vi "Begin.vi"(8 "error in":errorcluster) -> (0 "error out":errorcluster)   [LabVIEW 2016]
doc: "Called before other user functions, this VI is expected to open initial I/O refnums, load in file data, and do all program initialization. Notice that the <B>error out</B> terminal is simply used for data flow. Wiring it to other structures or subVIs ensures that this VI runs first."
uses:
  <vilib>/Rock Robotics/WPI/DriverStation/WPI_DriverStationRobotMode2.ctl
  <vilib>/Rock Robotics/WPI/Joystick/WPI_JoystickDeviceEnum.ctl
  <vilib>/Rock Robotics/WPI/ThirdParty/CanMotor/TalonSRX/WPI_CANTalonSRX_APIControlMode.ctl
  <vilib>/Rock Robotics/WPI/SafetyOutput/WPI_SafetyOutputConfigMenu.ctl
  <vilib>/Rock Robotics/SystemInterfaces/DIO/FPGA_DIOPWMChannel.ctl
  <vilib>/Rock Robotics/SystemInterfaces/DIO/FPGA_DIOChannel.ctl
  <vilib>/Rock Robotics/WPI/ThirdParty/CanMotor/TalonSRX/WPI_CANTalonSRX_Params.ctl
  Robot Global Data.vi
  <vilib>/Rock Robotics/Network Tables/NT Write String Array.vi
  <vilib>/Rock Robotics/WPI/MotorControl/WPI_MotorControlOpen TalonSRX.vi
  <vilib>/Rock Robotics/WPI/MotorControl/WPI_MotorControlOpen Talon.vi
  <vilib>/Rock Robotics/WPI/RobotDrive/WPI_RobotDriveOpen4MotorWithExistingMotors.vi
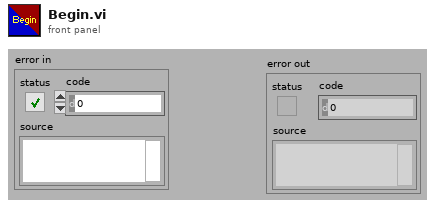
[diagram p1: front panel]
types:
  T1 = typedef "WPI_CANTalonSRX_Params.ctl" = u8
  T2 = typedef "WPI_CANTalonSRX_APIControlMode.ctl" = enum8{"Percent VBus", "Speed", "Position", "Slave", "Unchanged / Invalid", "Voltage Compensation", "Current", "Motion Profile", "Motion Magic"}
  T3 = typedef "FPGA_DIOPWMChannel.ctl" = enum8{"PWM 0", "PWM 1", "PWM 2", "PWM 3", "PWM 4", "PWM 5", "PWM 6", "PWM 7", "PWM 8", "PWM 9", "PWM MXP 0", "PWM MXP 1", "PWM MXP 2", "PWM MXP 3", "PWM MXP 4", "PWM MXP 5", "PWM MXP 6", "PWM MXP 7", "PWM MXP 8", "PWM MXP 9", "Invalid"}
  T4 = typedef "FPGA_DIOChannel.ctl" = enum8{"DIO 0", "DIO 1", "DIO 2", "DIO 3", "DIO 4", "DIO 5", "DIO 6", "DIO 7", "DIO 8", "DIO 9", "DIO MXP 0", "DIO MXP 1", "DIO MXP 2", "DIO MXP 3", "DIO MXP 4", "DIO MXP 5", "DIO MXP 6", "DIO MXP 7", "DIO MXP 8", "DIO MXP 9", "DIO MXP 10", "DIO MXP 11", "DIO MXP 12", "DIO MXP 13", "DIO MXP 14", "DIO MXP 15", "SPI Port CS1", "SPI Port CS2", "SPI Port CS3", "SPI Port MISO", "SPI Port MOSI", "Invalid"}
  T5 = typedef "WPI_JoystickDeviceEnum.ctl" = enum16{"USB 0", "USB 1", "USB 2", "USB 3", "USB 4", "USB 5"}
  T6 = typedef "WPI_SafetyOutputConfigMenu.ctl" = enum16{"Enable", "Disable"}
  T7 = typedef "WPI_DriverStationRobotMode2.ctl" = enum16{"Autonomous Disabled", "Autonomous Enabled", "Teleop Disabled", "Teleop Enabled", "Disconnected", "Finish", "Test Disabled", "Test Enabled", "Emergency Stopped"}
  T8 = typedef "WPI_DigitalInputDevRef.ctl" = cluster{"DevStatus":errorcluster, "DIO Channel":T4}
  T9 = typedef "WPI_MotorControlDeviceRef.ctl" = cluster{"DeviceStatus":errorcluster, "Type":T10, "PWM":cluster{"PWM Channel":T3, "DeadBand":T11}, "CAN":cluster{"Device Number":u8, "SetOutput VI Ref":variant, "GetOutput VI Ref":variant, "Enable VI Ref":variant, "Disable VI Ref":variant, "Data":variant}, "Invert":bool}
  T10 = typedef "WPI_MotorControlType.ctl" = enum16{"PWM", "CAN"}
  T11 = typedef "WPI_PWMDeadband.ctl" = cluster{"Name":string, "maxPositivePwm":i32, "minPositivePwm":i32, "centerPwm":i32, "maxNegativePwm":i32, "minNegativePwm":i32, "angularRange":u16}
  T12 = typedef "WPI_JoystickDevRef.ctl" = cluster{"Device":T5}
  T13 = typedef "WPI_RobotDriveDevRef.ctl" = cluster{"DevStatus":errorcluster, "Motors[]":T9[], "Square Inputs":bool, "Max Output":dbl}
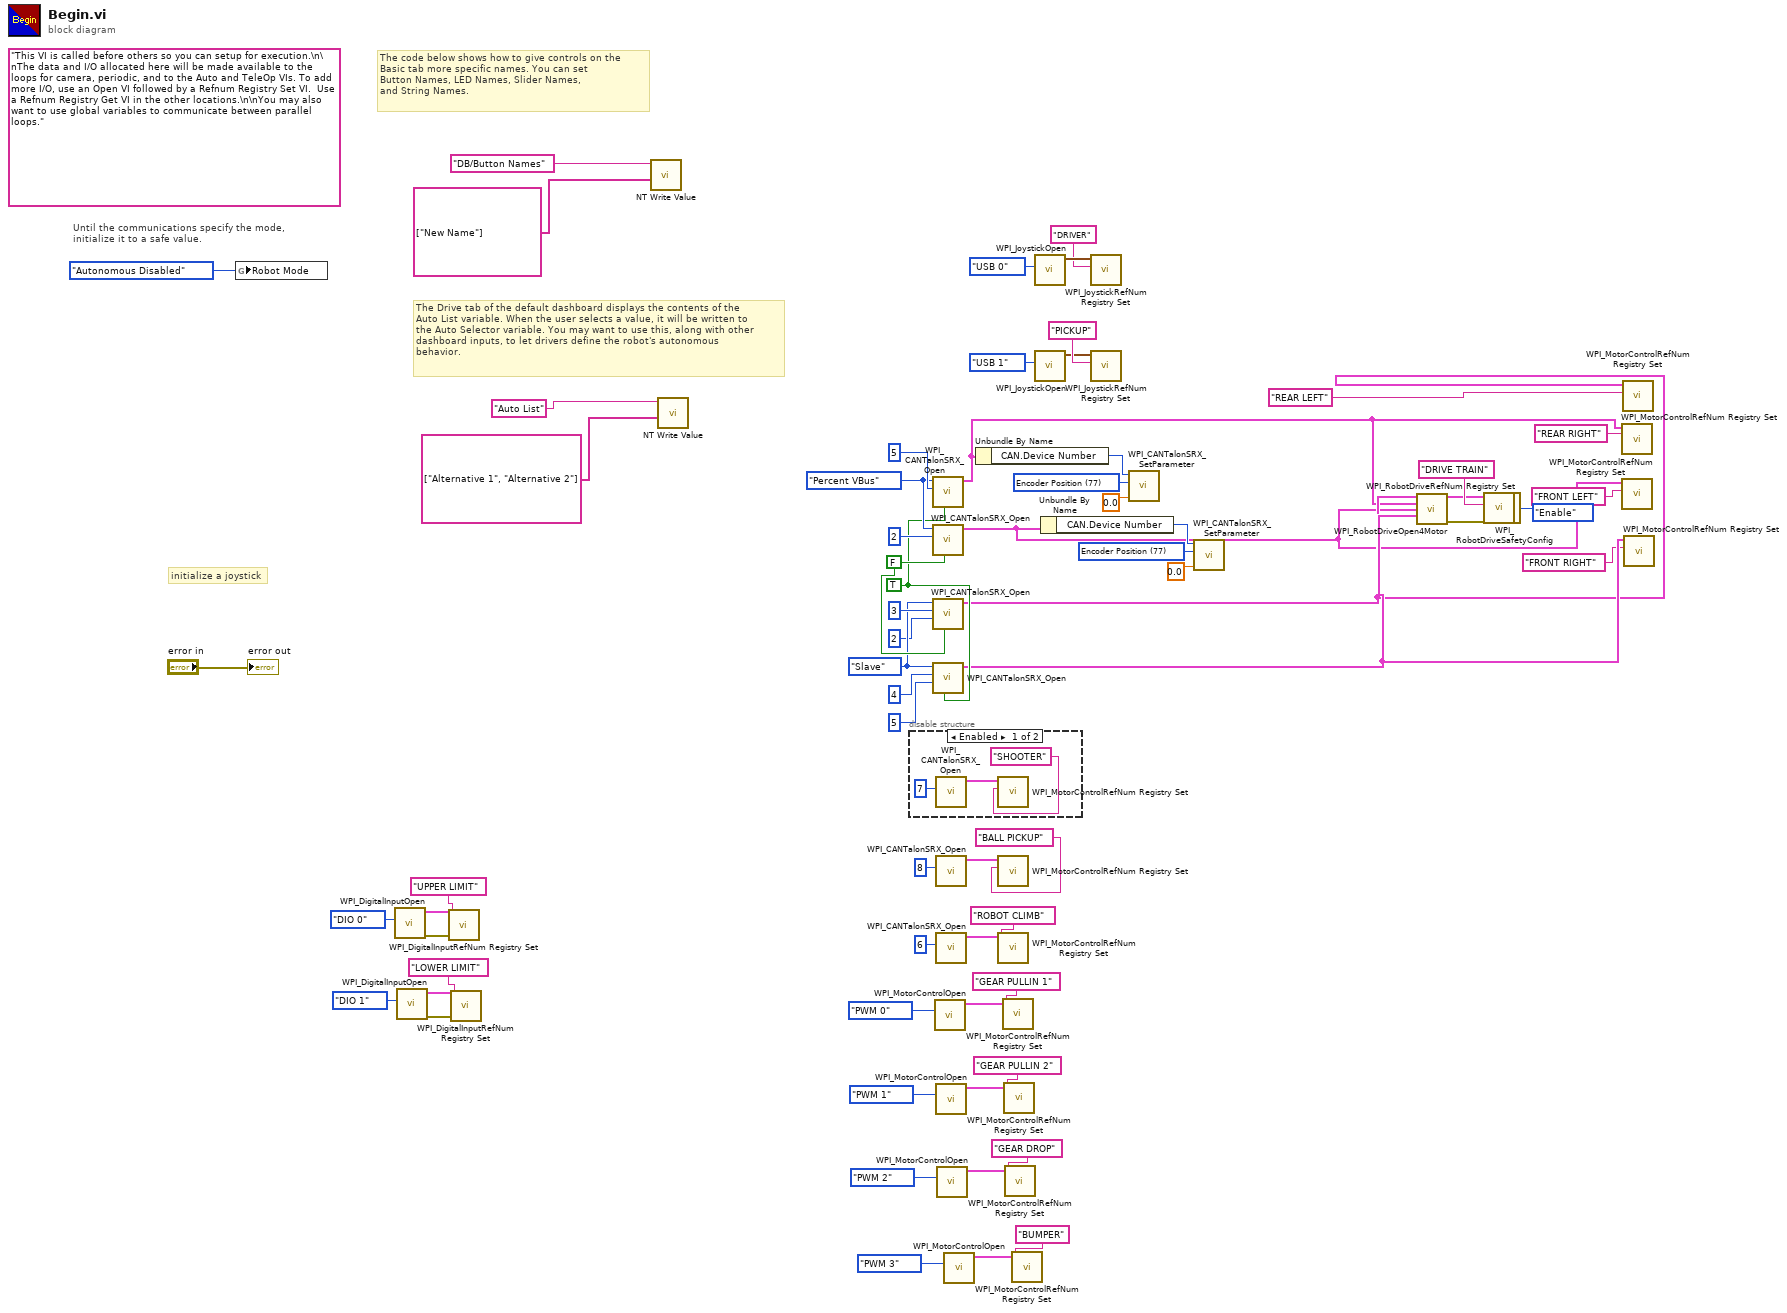
[diagram p0: block diagram]
diagram:
  w3 = T1 77 items=["Slot 0 - P"=1, "Slot 0 - I"=2, "Slot 0 - D"=3, "Slot 0 - F"=4, "Slot 0 - I Zone"=5, "Slot 0 - Ramp Rate"=6, "Slot 1 - P"=11, "Slot 1 - I"=12, "Slot 1 - D"=13, "Slot 1 - F"=14, "Slot 1 - I Zone"=15, "Slot 1 - Ramp Rate"=16, "Soft Limit - Forward"=21, "Soft Limit - Reverse"=22, "Soft Limit - Forward Enable"=23, "Soft Limit - Reverse Enable"=24, "On Boot - Brake Mode"=31, "On Boot - Limit Normally Closed - Forward"=32, "On Boot - Limit Normally Closed - Reverse"=33, "On Boot - Limit Disabled - Forward"=34, "On Boot - Limit Disabled - Reverse"=35, "Fault - Over Temp"=41, "Fault - Under Voltage"=42, "Fault - Forward Limit"=43, "Fault - Reverse Limit"=44, "Fault - Hardware Failure"=45, "Fault - Forward Soft Limit"=46, "Fault - Reverse Soft Limit"=47, "Sticky Fault - Over Temp"=48, "Sticky Fault - Under Voltage"=49, "Sticky Fault - Forward Limit"=50, "Sticky Fault - Reverse Limit"=51, "Sticky Fault - Forward Soft Limit"=52, "Sticky Fault - Reverse Soft Limit"=53, "Applied Throttle"=61, "Closed-Loop Error"=62, "Select Feedback Device"=63, "Reverse Closed-Loop Output"=64, "Mode Select"=65, "Profile Slot Select"=66, "Ramp Throttle"=67, "Reverse Feedback Sensor"=68, "Limit Switch Enabled"=69, "Limit Switch Closed - Forward"=70, "Limit Switch Closed - Reverse"=71, "Sensor Position"=73, "Sensor Velocity"=74, "Current"=75, "Brake is Enabled"=76, "Encoder Position"=77, "Encoder Velocity"=78, "Encoder Index Rise Events"=79, "Encoder A Pin State"=80, "Encoder B Pin State"=81, "Encoder Index Pin State"=82, "Analog In with Overflow"=83, "Analog In Velocity"=84, "Temperature"=85, "Battery Voltage"=86, "Reset Count"=87, "Reset Flags"=88, "Firmware Version"=89, "Settings Changed"=90, "Quad Filter Enable"=91, "Ignore Disable Broadcast"=92, "I Accumulator"=93, "Status 1 Frame Rate Ms"=94, "Status 2 Frame Rate Ms"=95, "Status 3 Frame Rate Ms"=96, "Status 4 Frame Rate Ms"=97, "Status 6 Frame Rate Ms"=98, "Status 7 Frame Rate Ms"=99, "Enable Index Pin Clear Position"=100, "Peak Positive Output"=104, "Nominal Positive Output"=105, "Peak Negative Output"=106, "Nominal Negative Output"=107, "Quad Index Pin Polarity"=108, "Status 8 Frame Rate Ms"=109, "Allow Position Overflow"=110, "Slot 0 - Allowable Closed-Loop Error"=111, "Number Potentiometer Turns"=112, "Encoder Codes Per Rev"=113, "Pulse Width Decoded Position"=114, "Analog Position"=115, "Voltage Compensation Rate (V/s)"=116, "Slot 1 - Allowable Closed-Loop Error"=117, "Motion Profile Has Underrun Err"=119, "Reserved 120"=120, "Legacy Control Mode"=121, "Motion Magic Acceleration"=122, "Motion Magic Cruise Velocity"=123, "Status 10 Frame Rate"=124, "Current Limit Threshold"=125, "CustomParam0"=137, "CustomParam1"=138, "PersStorageSaving"=139, "ClearPositionOnLimitF"=144, "ClearPositionOnLimitR"=145, "NominalBatteryVoltage"=146, "SampleVelocityPeriod"=147, "SampleVelocityWindow"=148] ("Parameter")
  w7 = T1 77 items=["Slot 0 - P"=1, "Slot 0 - I"=2, "Slot 0 - D"=3, "Slot 0 - F"=4, "Slot 0 - I Zone"=5, "Slot 0 - Ramp Rate"=6, "Slot 1 - P"=11, "Slot 1 - I"=12, "Slot 1 - D"=13, "Slot 1 - F"=14, "Slot 1 - I Zone"=15, "Slot 1 - Ramp Rate"=16, "Soft Limit - Forward"=21, "Soft Limit - Reverse"=22, "Soft Limit - Forward Enable"=23, "Soft Limit - Reverse Enable"=24, "On Boot - Brake Mode"=31, "On Boot - Limit Normally Closed - Forward"=32, "On Boot - Limit Normally Closed - Reverse"=33, "On Boot - Limit Disabled - Forward"=34, "On Boot - Limit Disabled - Reverse"=35, "Fault - Over Temp"=41, "Fault - Under Voltage"=42, "Fault - Forward Limit"=43, "Fault - Reverse Limit"=44, "Fault - Hardware Failure"=45, "Fault - Forward Soft Limit"=46, "Fault - Reverse Soft Limit"=47, "Sticky Fault - Over Temp"=48, "Sticky Fault - Under Voltage"=49, "Sticky Fault - Forward Limit"=50, "Sticky Fault - Reverse Limit"=51, "Sticky Fault - Forward Soft Limit"=52, "Sticky Fault - Reverse Soft Limit"=53, "Applied Throttle"=61, "Closed-Loop Error"=62, "Select Feedback Device"=63, "Reverse Closed-Loop Output"=64, "Mode Select"=65, "Profile Slot Select"=66, "Ramp Throttle"=67, "Reverse Feedback Sensor"=68, "Limit Switch Enabled"=69, "Limit Switch Closed - Forward"=70, "Limit Switch Closed - Reverse"=71, "Sensor Position"=73, "Sensor Velocity"=74, "Current"=75, "Brake is Enabled"=76, "Encoder Position"=77, "Encoder Velocity"=78, "Encoder Index Rise Events"=79, "Encoder A Pin State"=80, "Encoder B Pin State"=81, "Encoder Index Pin State"=82, "Analog In with Overflow"=83, "Analog In Velocity"=84, "Temperature"=85, "Battery Voltage"=86, "Reset Count"=87, "Reset Flags"=88, "Firmware Version"=89, "Settings Changed"=90, "Quad Filter Enable"=91, "Ignore Disable Broadcast"=92, "I Accumulator"=93, "Status 1 Frame Rate Ms"=94, "Status 2 Frame Rate Ms"=95, "Status 3 Frame Rate Ms"=96, "Status 4 Frame Rate Ms"=97, "Status 6 Frame Rate Ms"=98, "Status 7 Frame Rate Ms"=99, "Enable Index Pin Clear Position"=100, "Peak Positive Output"=104, "Nominal Positive Output"=105, "Peak Negative Output"=106, "Nominal Negative Output"=107, "Quad Index Pin Polarity"=108, "Status 8 Frame Rate Ms"=109, "Allow Position Overflow"=110, "Slot 0 - Allowable Closed-Loop Error"=111, "Number Potentiometer Turns"=112, "Encoder Codes Per Rev"=113, "Pulse Width Decoded Position"=114, "Analog Position"=115, "Voltage Compensation Rate (V/s)"=116, "Slot 1 - Allowable Closed-Loop Error"=117, "Motion Profile Has Underrun Err"=119, "Reserved 120"=120, "Legacy Control Mode"=121, "Motion Magic Acceleration"=122, "Motion Magic Cruise Velocity"=123, "Status 10 Frame Rate"=124, "Current Limit Threshold"=125, "CustomParam0"=137, "CustomParam1"=138, "PersStorageSaving"=139, "ClearPositionOnLimitF"=144, "ClearPositionOnLimitR"=145, "NominalBatteryVoltage"=146, "SampleVelocityPeriod"=147, "SampleVelocityWindow"=148] ("Parameter")
  w11 = WPI_CANTalonSRX_APIControlMode."Slave" ("Control Mode")
  w49 = TRUE ("Invert")
  w50 = FALSE ("Invert")
  w54 = WPI_CANTalonSRX_APIControlMode."Percent VBus" ("Control Mode")
  (unwired) "This VI is called before others so you can setup for execution.\n\nThe data and I/O allocated here will be made available to the loops for camera, periodic, and to the Auto and TeleOp VIs. To add more I/O, use an Open VI followed by a Refnum Registry Set VI.  Use a Refnum Registry Get VI in the other locations.\n\nYou may also want to use global variables to communicate between parallel loops."
  # "The Drive tab of the default dashboard displays the contents of the\nAuto List variable. When the user selects a value, it will be written to\nthe Auto Selector variable. You may want to use this, along with other\ndashboard inputs, to let drivers define the robot's autonomous\nbehavior."
  # "The code below shows how to give controls on the\nBasic tab more specific names. You can set\nButton Names, LED Names, Slider Names,\nand String Names."
  # "initialize a joystick"
  # "Until the communications specify the mode,\ninitialize it to a safe value."
  n1 = global write "Robot Global Data.vi" "Robot Mode"(WPI_DriverStationRobotMode2."Autonomous Disabled" ("Robot Mode")) -> ()
  n2 = call <vilib>:"WPI_DigitalInputOpen.vi"("DIO Channel"=FPGA_DIOChannel."DIO 0") -> ("error out"=w22:errorcluster, "DigitalInputDevRef"=w21:T8)  [unwired: 9 in]
  n3 = call <vilib>:"WPI_DigitalInputOpen.vi"("DIO Channel"=FPGA_DIOChannel."DIO 1") -> ("error out"=w15:errorcluster, "DigitalInputDevRef"=w16:T8)  [unwired: 9 in]
  n4 = call <vilib>:"WPI_DigitalInputRefNum Registry Set.vi"("error in (no error)"=w22, "refnum name"="UPPER LIMIT", "DigitalInputDevRef"=w21) -> ()  [unwired: 7 in, 2 out]
  n5 = call <vilib>:"WPI_DigitalInputRefNum Registry Set.vi"("error in (no error)"=w15, "refnum name"="LOWER LIMIT", "DigitalInputDevRef"=w16) -> ()  [unwired: 7 in, 2 out]
  n6 = call-poly <vilib>:"NT Write Value.vi"("String Array"=string[] ["New Name"], "Name"="DB/Button Names") -> ()  [unwired: 9 in, 1 out]
  n7 = call-poly <vilib>:"NT Write Value.vi"("String Array"=string[] ["Alternative 1", "Alternative 2"], "Name"="Auto List") -> ()  [unwired: 9 in, 1 out]
  n8 = disable-structure shown="Enabled" {
    frame Enabled {
      n9 = call <vilib>:"WPI_CANTalonSRX_Open.vi"("Device Number"=u8 7) -> ("CAN Talon SRX Ref"=w69:T9)  [unwired: 9 in, 1 out]
      n10 = call <vilib>:"WPI_MotorControlRefNum Registry Set.vi"("refnum name"="SHOOTER", "MotorControlDevRef"=w69) -> ()  [unwired: 8 in, 2 out]
    }
    frame Disabled {
    }
  }
  n11 = call <vilib>:"WPI_CANTalonSRX_Open.vi"("Invert"=w49, "Device Number"=u8 5, "Control Mode"=w54) -> ("CAN Talon SRX Ref"=w1:T9)  [unwired: 7 in, 1 out]
  n12 = call <vilib>:"WPI_CANTalonSRX_Open.vi"("Invert"=w50, "Device Number"=u8 2, "Control Mode"=w54) -> ("CAN Talon SRX Ref"=w5:T9)  [unwired: 7 in, 1 out]
  n13 = call <vilib>:"WPI_CANTalonSRX_Open.vi"("Invert"=w50, "Master Device Number"=u8 2, "Device Number"=u8 3, "Control Mode"=w11) -> ("CAN Talon SRX Ref"=w27:T9)  [unwired: 6 in, 1 out]
  n14 = call <vilib>:"WPI_CANTalonSRX_Open.vi"("Invert"=w49, "Master Device Number"=u8 5, "Device Number"=u8 4, "Control Mode"=w11) -> ("CAN Talon SRX Ref"=w28:T9)  [unwired: 6 in, 1 out]
  n15 = call-poly <vilib>:"WPI_MotorControlOpen.vi"("PWM Channel"=FPGA_DIOPWMChannel."PWM 0") -> ("MotorControlDeviceRef"=w35:T9)  [unwired: 9 in, 1 out]
  n16 = call <vilib>:"WPI_CANTalonSRX_Open.vi"("Device Number"=u8 8) -> ("CAN Talon SRX Ref"=w43:T9)  [unwired: 9 in, 1 out]
  n17 = call <vilib>:"WPI_CANTalonSRX_Open.vi"("Device Number"=u8 6) -> ("CAN Talon SRX Ref"=w40:T9)  [unwired: 9 in, 1 out]
  n18 = call-poly <vilib>:"WPI_MotorControlOpen.vi"("PWM Channel"=FPGA_DIOPWMChannel."PWM 1") -> ("MotorControlDeviceRef"=w34:T9)  [unwired: 9 in, 1 out]
  n19 = call-poly <vilib>:"WPI_MotorControlOpen.vi"("PWM Channel"=FPGA_DIOPWMChannel."PWM 2") -> ("MotorControlDeviceRef"=w29:T9)  [unwired: 9 in, 1 out]
  n20 = call-poly <vilib>:"WPI_MotorControlOpen.vi"("PWM Channel"=FPGA_DIOPWMChannel."PWM 3") -> ("MotorControlDeviceRef"=w14:T9)  [unwired: 9 in, 1 out]
  n21 = Unbundle By Name(w1) -> ("CAN.Device Number"=w4:u8)
  n22 = call <vilib>:"WPI_MotorControlRefNum Registry Set.vi"("refnum name"="BALL PICKUP", "MotorControlDevRef"=w43) -> ()  [unwired: 8 in, 2 out]
  n23 = call <vilib>:"WPI_MotorControlRefNum Registry Set.vi"("refnum name"="ROBOT CLIMB", "MotorControlDevRef"=w40) -> ()  [unwired: 8 in, 2 out]
  n24 = call <vilib>:"WPI_MotorControlRefNum Registry Set.vi"("refnum name"="GEAR PULLIN 1", "MotorControlDevRef"=w35) -> ()  [unwired: 8 in, 2 out]
  n25 = call <vilib>:"WPI_MotorControlRefNum Registry Set.vi"("refnum name"="GEAR PULLIN 2", "MotorControlDevRef"=w34) -> ()  [unwired: 8 in, 2 out]
  n26 = call <vilib>:"WPI_MotorControlRefNum Registry Set.vi"("refnum name"="GEAR DROP", "MotorControlDevRef"=w29) -> ()  [unwired: 8 in, 2 out]
  n27 = call <vilib>:"WPI_MotorControlRefNum Registry Set.vi"("refnum name"="BUMPER", "MotorControlDevRef"=w14) -> ()  [unwired: 8 in, 2 out]
  n28 = call <vilib>:"WPI_JoystickOpen.vi"("JoystickDevice"=WPI_JoystickDeviceEnum."USB 0") -> ("JoystickDevRef"=w46:T12)  [unwired: 10 in]
  n29 = call <vilib>:"WPI_JoystickOpen.vi"("JoystickDevice"=WPI_JoystickDeviceEnum."USB 1") -> ("JoystickDevRef"=w65:T12)  [unwired: 10 in]
  n30 = Unbundle By Name(w5) -> ("CAN.Device Number"=w8:u8)
  n31 = call <vilib>:"WPI_JoystickRefNum Registry Set.vi"("refnum name"="DRIVER", "JoystickDevRef"=w46) -> ()  [unwired: 8 in, 2 out]
  n32 = call <vilib>:"WPI_JoystickRefNum Registry Set.vi"("refnum name"="PICKUP", "JoystickDevRef"=w65) -> ()  [unwired: 8 in, 2 out]
  n33 = call <vilib>:"WPI_CANTalonSRX_SetParameter.vi"("Value"=0.0, "Parameter"=w3, "Device ID (0)"=w4) -> ()  [unwired: 7 in, 2 out]
  n34 = call <vilib>:"WPI_CANTalonSRX_SetParameter.vi"("Value"=0.0, "Parameter"=w7, "Device ID (0)"=w8) -> ()  [unwired: 7 in, 2 out]
  n35 = call-poly <vilib>:"WPI_RobotDriveOpen4Motor.vi"("Rear Left Motor Dev Ref"=w27, "Rear Right Motor Dev Ref"=w1, "Front Left Motor Dev Ref"=w5, "Front Right Motor Dev Ref"=w28) -> ("RobotDriveDevRef"=w48:T13, "error out"=w44:errorcluster)  [unwired: 10 in]
  n36 = call <vilib>:"WPI_RobotDriveRefNum Registry Set.vi"("error in (no error)"=w44, "refnum name"="DRIVE TRAIN", "RobotDriveDevRef"=w48) -> ("RobotDriveDevRef"=w52:T13)  [unwired: 1 in, 7 out]
  n37 = call <vilib>:"WPI_RobotDriveSafetyConfig.vi"("mode"=WPI_SafetyOutputConfigMenu."Enable", "RobotDriveDevRef"=w52) -> ()  [unwired: 8 in, 2 out]
  n38 = call <vilib>:"WPI_MotorControlRefNum Registry Set.vi"("refnum name"="REAR RIGHT", "MotorControlDevRef"=w1) -> ()  [unwired: 8 in, 2 out]
  n39 = call <vilib>:"WPI_MotorControlRefNum Registry Set.vi"("refnum name"="FRONT LEFT", "MotorControlDevRef"=w5) -> ()  [unwired: 8 in, 2 out]
  n40 = call <vilib>:"WPI_MotorControlRefNum Registry Set.vi"("refnum name"="REAR LEFT", "MotorControlDevRef"=w27) -> ()  [unwired: 8 in, 2 out]
  n41 = call <vilib>:"WPI_MotorControlRefNum Registry Set.vi"("refnum name"="FRONT RIGHT", "MotorControlDevRef"=w28) -> ()  [unwired: 8 in, 2 out]
  "error out" <- "error in"
